vi "Error Engine Stop.vi"(8 "error in (no error)":errorcluster) -> (0 "error out":errorcluster)   [LabVIEW 2023, in "HardwareAbstractionLayer_LVOOP.lvlib" / "Error Handler.lvclass"]
uses:
  Error Handler.lvclass
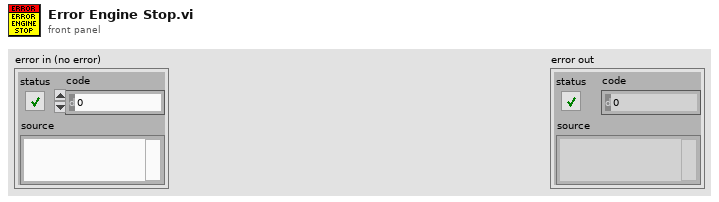
[diagram p1: front panel]
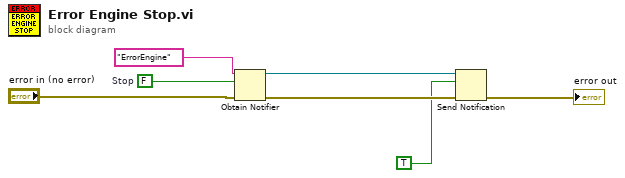
[diagram p0: block diagram]
diagram:
  w7 = FALSE  # Stop
  n1 = Obtain Notifier(name (unnamed)="ErrorEngine", notification data type=w7, error in (no error)="error in (no error)") -> (notifier out=w4:refnum<notifier>, error out=w3:errorcluster)  [unwired: 1 in, 1 out]
  n2 = Send Notification(notification=TRUE, notifier=w4, error in (no error)=w3) -> (error out=→"error out":errorcluster)  [unwired: 1 out]
